vi "query logic.vi"(7 "type":enum16{"selector", "send"}(ring)=enum."send", 10 "OldVal":T1[](array[typedef]), 11 "NewVal":T1[](array[typedef])) -> (1 "selector":string, 2 "Numeric":i32, 3 "NewVal  OUT":T1[](array[typedef]))   [LabVIEW 2014]
uses:
  query.ctl
panel:
  in  "misc controls":refnum<vi>
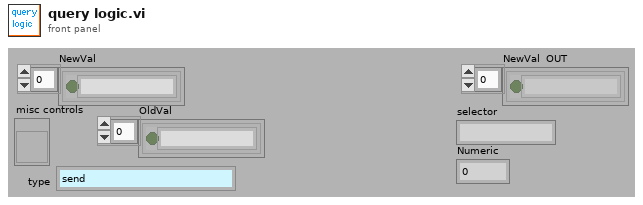
[diagram p1: front panel]
types:
  T1 = typedef "query.ctl" = cluster{"Boolean":bool, "String":string}
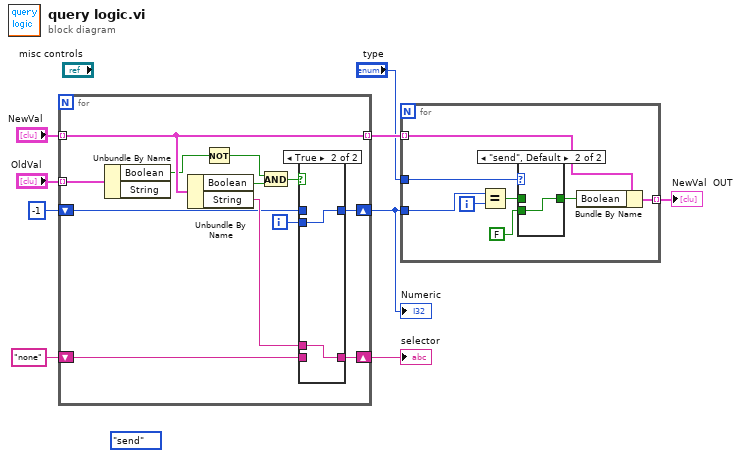
[diagram p0: block diagram]
diagram:
  (unwired) enum16{"selector", "send"}."send" ("type")
  n1 = for {
    tunnel: "NewVal" -> [w18] mode=indexing
    shift-right: [w21] -> w8
    shift-left: "none" -> [w19]
    tunnel: [w18] -> w6 mode=indexing
    shift-right: [w17] -> w3
    shift-left: -1 -> [w15]
    tunnel: "OldVal" -> [w14] mode=indexing
    i -> [w16]
    n2 = Unbundle By Name(w14) -> ("Boolean"=w13:bool)  [unwired: 1 out]
    n3 = Unbundle By Name(w18) -> ("Boolean"=w11:bool, "String"=w20:string)
    n4 = Not(x=w13) -> (.not. x?=w12:bool)
    n5 = And(x=w12, y=w11) -> (x .and. y?=w10:bool)
    n6 = case shown="True" w10 {
      tunnel: [w23 w25] -> w21
      tunnel: w20 -> [_ w25]
      tunnel: w19 -> [w23 _]
      tunnel: [w22 w24] -> w17
      tunnel: w16 -> [_ w24]
      tunnel: w15 -> [w22 _]
      frame False {
      }
      frame True {
      }
    }
  }
  "selector" <- w8
  "Numeric" <- w3
  n7 = for {
    tunnel: w6 -> [w33] mode=indexing
    tunnel: [w32] -> w5 mode=indexing
    tunnel: w3 -> [w30]
    tunnel: "type" -> [w29]
    i -> [w31]
    n8 = Equal?(x=w30, y=w31) -> (x = y?=w26:bool)
    n9 = case shown="\"send\", Default" w29 {
      tunnel: [w34 w35] -> w28
      tunnel: FALSE -> [_ w35]
      tunnel: w26 -> [w34 _]
      frame "selector" {
      }
      frame "send", Default {
      }
    }
    n10 = Bundle By Name(cluster=w33, "Boolean"=w28) -> (w32:T1)
  }
  "NewVal  OUT" <- w5
